vi "Zotero Export.vi"() -> ()   [LabVIEW 2021]
uses:
  <vilib>/httpClient/LabVIEWHTTPClient.lvlib
  ARKEO_win/PPL/JSONtext.lvlibp
panel:
  in  "index":i32
  out "<JSON>":string caption="<JSON>First JSON Value"
  out "headers":string
  out "body":string
  out "error out":errorcluster
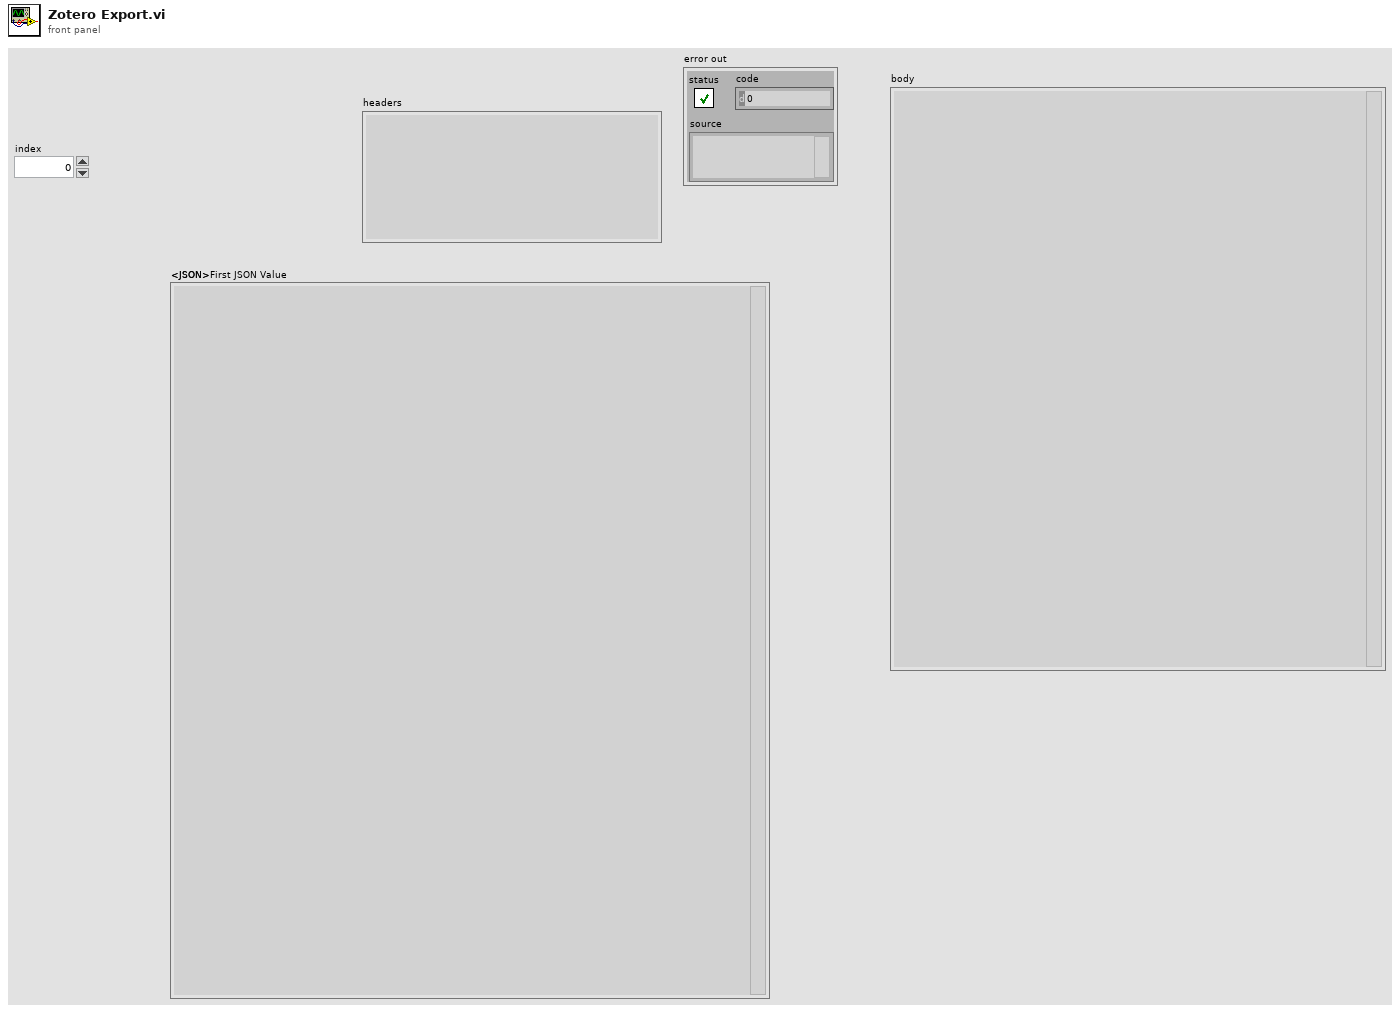
[diagram p1: front panel]
types:
  T1 = typedef "LabVIEWHTTPClient.lvlib/ClientHandle.ctl" = refnum<k1>
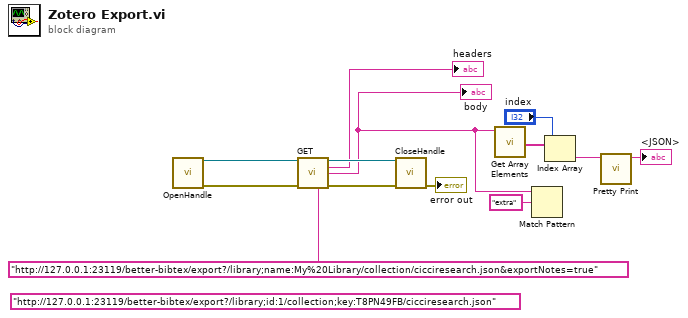
[diagram p0: block diagram]
diagram:
  (unwired) "http://127.0.0.1:23119/better-bibtex/export?/library;id:1/collection;key:T8PN49FB/cicciresearch.json"
  n1 = call <vilib>:"OpenHandle.vi"() -> ("client handle out"=w13:T1, "error out"=w12:errorcluster)  [unwired: 14 in]
  n2 = call <vilib>:"GET.vi"("client handle"=w13, "url"="http://127.0.0.1:23119/better-bibtex/export?/library;name:My%20Library/collection/cicciresearch.json&exportNotes=true", "error in (no error)"=w12) -> ("client handle out"=w11:T1, "headers"=→"headers":string, "body"=w2:string, "error out"=w10:errorcluster)  [unwired: 9 in]
  "body" <- w2
  n3 = call <vilib>:"CloseHandle.vi"("client handle"=w11, "error in (no error)"=w10) -> ("error out"=→"error out":errorcluster)  [unwired: 13 in]
  n4 = call "Get Array Elements.vi"("JSON"=w2) -> ("<JSON>"=w6:string[])  [unwired: 8 in, 2 out]
  n5 = Match Pattern(string=w2, regular expression="extra") -> ()  [unwired: 1 in, 4 out]
  n6 = Index Array(array=w6, index="index") -> (element=w5:string)
  n7 = call "Pretty Print.vi"("JSON"=w5) -> ("<JSON>"=→"<JSON>":string)  [unwired: 8 in, 2 out]
